vi "Robotics_Module_Test.vi"() -> ()   [LabVIEW 2014]
uses:
  <vilib>/robotics/Kinematics/Analytical/NI_Robotics_AnalyticKinematics.lvlib
  <vilib>/robotics/Kinematics/Robot/NI_Robotics_Serial Robot Arm.lvclass
  <vilib>/robotics/Kinematics/NI_Kinematics.lvlib
  <vilib>/robotics/Kinematics/Generate Joint Trajectory (Int).vi
  <vilib>/Analysis/Matrix/Datatypes/RealMatrix.ctl
  <vilib>/Analysis/Matrix/NI_Matrix.lvlib
  <vilib>/robotics/Kinematics/Analytical/5R/Type 1/Initialize 5R Type 1 Serial Arm.vi
  <vilib>/robotics/Kinematics/Analytical/5R/Type 1/NI_Robotics_5R Type 1 Serial Arm Class.lvclass
  <vilib>/robotics/Kinematics/Plotting/NI_Robotics_3DKinematics.lvlib
  <vilib>/robotics/Kinematics/Robot/Robot Pose.ctl
panel:
  out "serial arm poses":T1[](array[typedef])
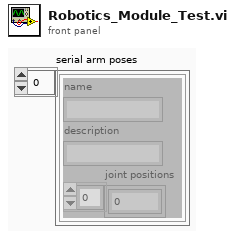
[diagram p1: front panel]
types:
  T1 = typedef "NI_Robotics_Serial Robot Arm.lvclass/Robot Pose.ctl" = cluster{"name":string, "description":string, "joint positions":dbl[]}
  T2 = typedef "NI_Matrix.lvlib/RealMatrix.ctl" = dbl[][]
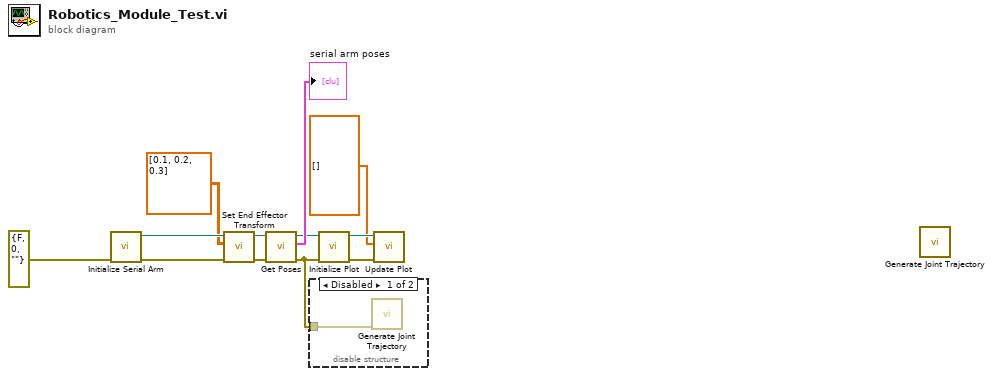
[diagram p0: block diagram]
diagram:
  n1 = call-poly <vilib>:"Initialize Serial Arm.vi"("error in (no error)"=errorcluster {"status"=FALSE, "code"=0, "source"=""}) -> ("error out"=w11:errorcluster, "5R type 1 serial arm out"=w12:refnum<class "NI_Robotics_5R Type 1 Serial Arm Class.lvclass">)  [unwired: 9 in]
  n2 = call <vilib>:"Set End Effector Transform.vi"("error in (no error)"=w11, "end effector transform"=T2 [[0.1], [0.2], [0.3]], "serial arm in"=w12) -> ("error out"=w9:errorcluster, "serial arm out"=w10:refnum<class "NI_Robotics_5R Type 1 Serial Arm Class.lvclass">)  [unwired: 7 in]
  n3 = call <vilib>:"Get Poses.vi"("error in (no error)"=w9, "serial arm in"=w10) -> ("error out"=w4:errorcluster, "serial arm poses"=→"serial arm poses":T1[], "serial arm out"=w5:refnum<class "NI_Robotics_5R Type 1 Serial Arm Class.lvclass">)  [unwired: 7 in]
  n4 = disable-structure shown="Disabled" {
    disable-tunnel: w4 -> [w13 _]
    frame Disabled {
      n5 = call-poly <vilib>:"Generate Joint Trajectory.vi"("error in (no error)"=w13) -> ()  [unwired: 7 in, 4 out]
    }
    frame Enabled {
    }
  }
  n6 = call <vilib>:"Initialize Plot.vi"("error in (no error)"=w4, "serial arm in"=w5) -> ("error out"=w1:errorcluster, "serial arm out"=w3:refnum<class "NI_Robotics_5R Type 1 Serial Arm Class.lvclass">)  [unwired: 8 in]
  n7 = call <vilib>:"Update Plot.vi"("error in (no error)"=w1, "joint positions"=dbl[] [], "serial arm in"=w3) -> ()  [unwired: 6 in, 3 out]
  n8 = call-poly <vilib>:"Generate Joint Trajectory.vi"() -> ()  [unwired: 8 in, 4 out]
